vi "VI Server_Set Signaling Control Value from String Format_ArrayInput.vi"(6 "Options":T1, 8 "error in (no error)":errorcluster, 9 "Values":string[](array[string]), 10 "Labels":string[](array[string]), 11 "VI Server Cluster":T2={"Labels"=["Label", "Size", "Font", "Heght", "Width", "Ledding Denominator", "Ledding Nominator", "Label Number", "Microstep Resolution", "X", "Y", "Z", "Italic?", "Underlined?"], "Refs"=[], "VI Ref"=refnum}) -> (0 "error out":errorcluster, 3 "VI Server Cluster.DUP":T2={"Labels"=["Label", "Size", "Font", "Heght", "Width", "Ledding Denominator", "Ledding Nominator", "Label Number", "Microstep Resolution", "X", "Y", "Z", "Italic?", "Underlined?"], "Refs"=[], "VI Ref"=refnum}, 5 "FailedLabel":string)   [LabVIEW 2020]
doc: "<B>Set Control Values From String Formats.vi</B> and converts string values of the selected GUI objects onto original data type."
uses:
  VI Server_TypeDefs/VI Server_RefsCluster.ctl
  VI Server Libraries/VI Server Controls.llb/VI Server_GetSet Controls From String Format_Options.ctl
  <vilib>/userDefined/High Color/IMAQdx.ctl
  VI Server Toolkit LV2013.lvlib
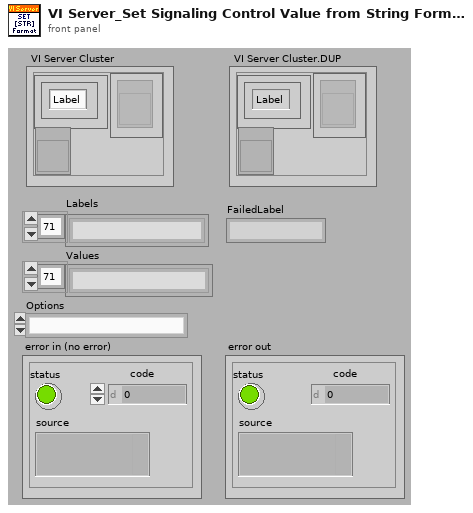
[diagram p1: front panel]
types:
  T1 = typedef "VI Server Toolkit LV2013.lvlib/VI Server_GetSet Controls From String Format_Options.ctl" = enum16{"", "If Ring Get Selection", "If Ring Set by Selection"}
  T2 = typedef "VI Server_RefsCluster.ctl" = cluster{"Labels":string[], "Refs":refnum<vi>[], "VI Ref":refnum<vi>}
  T3 = typedef "IMAQdx.ctl" = refnum<k21>
  T4 = typedef "LVStringsAndValuesArrayTypeDef_U32.ctl" = cluster{"String":string, "Value":u32}[]
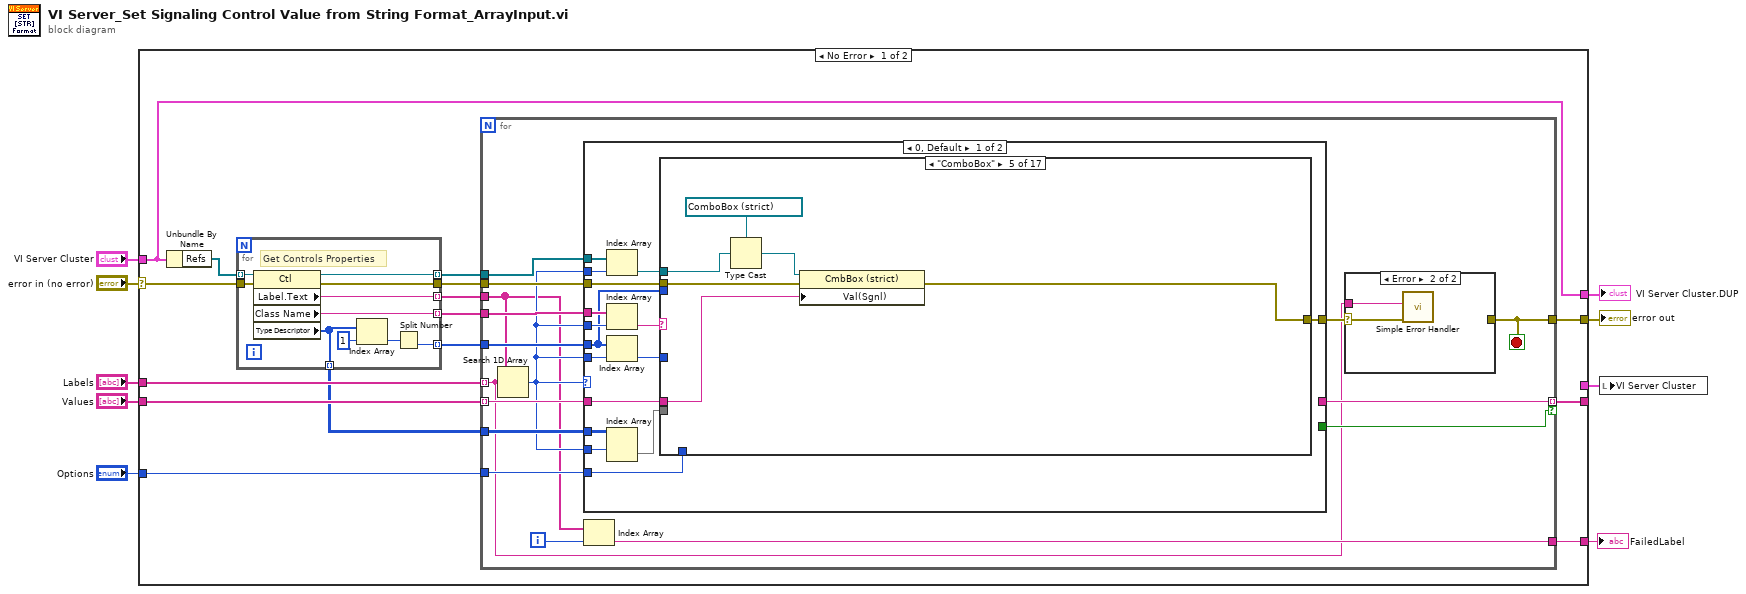
[diagram p0: block diagram]
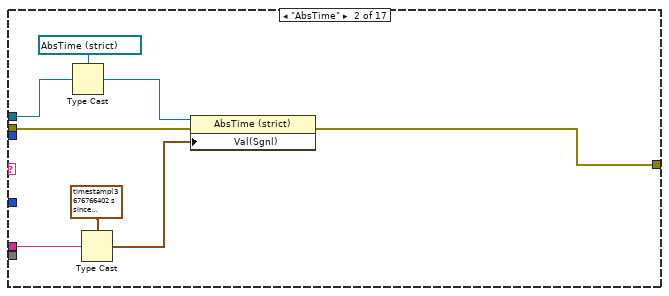
[diagram p4: hidden frame]
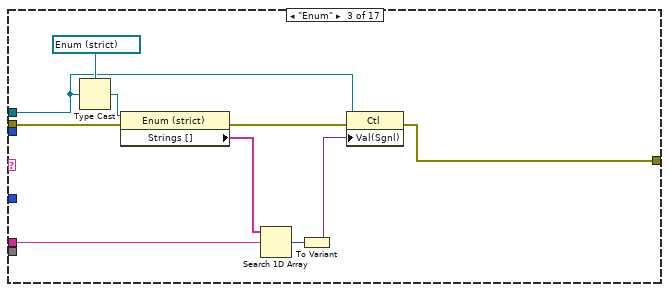
[diagram p5: hidden frame]
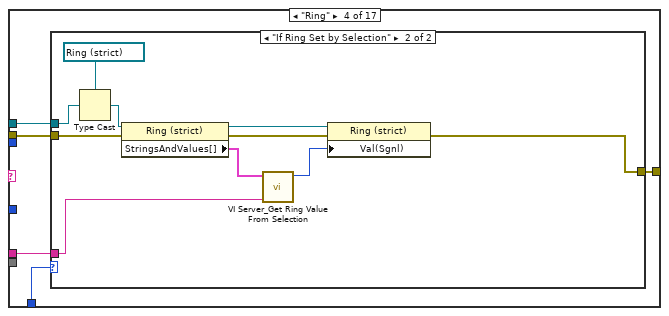
[diagram p6: hidden frame]
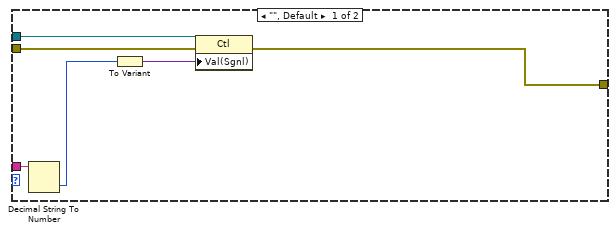
[diagram p7: hidden frame]
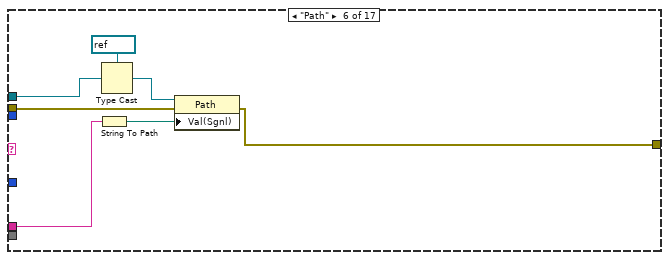
[diagram p8: hidden frame]
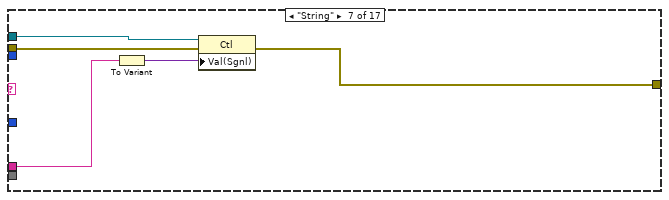
[diagram p9: hidden frame]
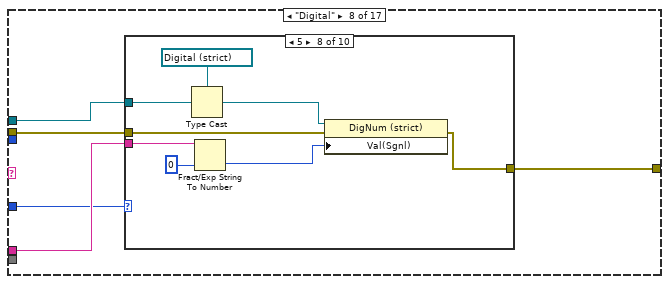
[diagram p10: hidden frame]
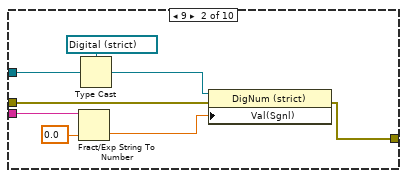
[diagram p12: hidden frame]
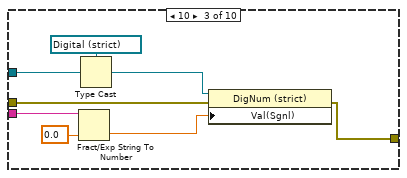
[diagram p13: hidden frame]
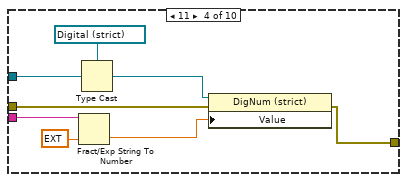
[diagram p14: hidden frame]
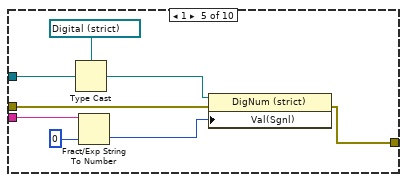
[diagram p15: hidden frame]
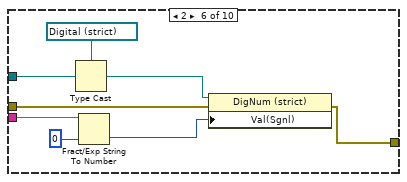
[diagram p16: hidden frame]
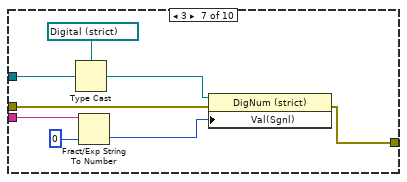
[diagram p17: hidden frame]
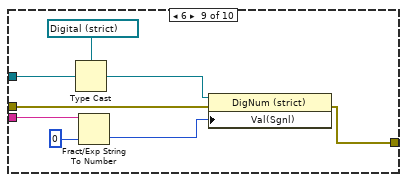
[diagram p18: hidden frame]
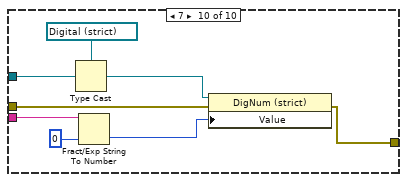
[diagram p19: hidden frame]
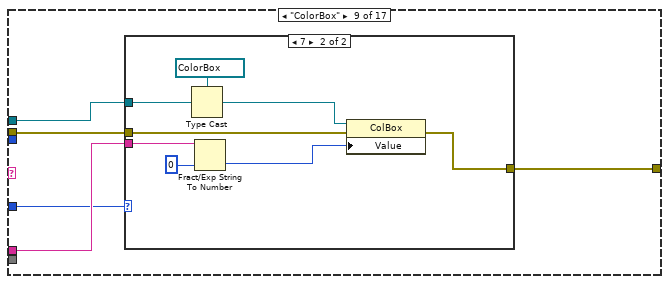
[diagram p20: hidden frame]
diagram:
  n1 = case shown="No Error" "error in (no error)" {
    selector: "error in (no error)" -> [w14 w631]
    tunnel: "Labels" -> [w19 _]
    tunnel: "Values" -> [w20 _]
    tunnel: [w13 w631] -> w7
    tunnel: [w12 _] -> w5
    tunnel: "VI Server Cluster" -> [w12 _]
    tunnel: "Options" -> [w15 _]
    tunnel: [_ w630] -> w2
    tunnel: [w11 _] -> _
    tunnel: [w10 _] -> w1
    frame No Error {
      n2 = Unbundle By Name(w12) -> ("Refs"=w18:refnum<vi>[])
      n3 = for {
        tunnel: w18 -> [w629] mode=indexing
        tunnel: w14 -> [w628]
        tunnel: [w627] -> w24 mode=indexing
        tunnel: [w626] -> w22 mode=indexing
        tunnel: [w625] -> w23 mode=indexing
        tunnel: [w624] -> w21
        tunnel: [w621] -> w17 mode=indexing
        tunnel: [w620] -> w16 mode=indexing
        # "Get Controls Properties"
        n4 = property class="Ctl"(reference=w629, error in=w628) -> (reference out=w625:refnum<vi>, error out=w624:errorcluster, "Label.Text"=w627:string, "Class Name"=w626:string, "Type Descriptor"=w620:i16[])
        n5 = Index Array(array=w620, index=1) -> (element=w622:i16)
        n6 = Split Number(x=w622) -> (lo(x)=w621:u8)  [unwired: 1 out]
      }
      n7 = for {
        tunnel: w19 -> [w25] mode=indexing
        tunnel: w24 -> [w30]
        tunnel: w23 -> [w38]
        tunnel: w22 -> [w40]
        tunnel: w20 -> [w39] mode=indexing
        tunnel: w21 -> [w37]
        tunnel: [w26] -> w13
        tunnel: w17 -> [w36]
        tunnel: w16 -> [w35]
        tunnel: w15 -> [w33]
        tunnel: [w32] -> w11 mode=indexing if=w31
        tunnel: [w28] -> w10
        i -> [w29]
        stop <- w26 stop-if-true
        n8 = Search 1D Array(1D array=w30, element=w25) -> (index of element=w34:i32)  [unwired: 1 out]
        n9 = case shown="0, Default" w34 {
          tunnel: w38 -> [w59 _]
          tunnel: w34 -> [w58 _]
          tunnel: w40 -> [w57 _]
          tunnel: w34 -> [w56 _]
          tunnel: w39 -> [w53 w618]
          tunnel: w37 -> [w52 w619]
          tunnel: [w51 w619] -> w27
          tunnel: w36 -> [w48 _]
          tunnel: w34 -> [w50 _]
          tunnel: w35 -> [w46 _]
          tunnel: w34 -> [w47 _]
          tunnel: w33 -> [w44 _]
          tunnel: [_ w618] -> w32
          tunnel: [_ TRUE] -> w31
          frame 0, Default {
            n10 = Index Array(array=w59, index=w58) -> (element=w54:refnum<vi>)
            n11 = Index Array(array=w57, index=w56) -> (element=w55:string)
            n12 = Index Array(array=w48, index=w50) -> (element=w49:u8)
            n13 = Index Array(array=w46, index (row)=w47) -> (element=w45:i16[])  [unwired: 1 in]
            n14 = case shown="\"ComboBox\"" w55 {
              tunnel: w54 -> [_ w68 w71 w80 w103 w108 w117 w120 w198 w212 w302 w309 w316 w488 w510 w531 w537]
              tunnel: w53 -> [_ w66 w76 w83 w100 w111 w115 w119 w197 w211 w295 w307 w315 w486 w511 w532 w538]
              tunnel: w52 -> [w60 w64 w74 w82 w105 w109 w114 w122 w200 w214 w304 w310 w320 w490 w512 w526 w539]
              tunnel: [w60 w63 w72 w81 w104 w110 w113 w121 w199 w213 w303 w305 w319 w489 w509 w529 w536] -> w51
              tunnel: w49 -> [_ _ _ _ _ _ _ w118 w196 w210 _ _ _ w487 _ _ _]
              tunnel: w48 -> [_ _ _ _ _ _ _ _ _ _ _ _ _ _ _ _ _]
              tunnel: w45 -> [_ _ _ _ _ _ _ _ _ _ _ _ w318 _ _ _ w535]
              tunnel: w44 -> [_ _ _ w79 _ _ _ _ _ _ _ _ _ _ _ _ _]
              frame "", Default {
              }
              frame "AbsTime" {
                n15 = Type Cast(type=refnum<vi> refnum ("UtilizationData.From"), x=w68) -> (*(type *) &x=w62:refnum<vi>)
                n16 = Type Cast(type=timestamp(3676766402.6552744 s since 1904-01-01) ("UtilizationData.From"), x=w66) -> (*(type *) &x=w61:timestamp)
                n17 = property class="AbsTime (strict)"(reference=w62, error in=w64, "Val(Sgnl)"=w61) -> (error out=w63:errorcluster)  [unwired: 1 out]
              }
              frame "Enum" {
                n18 = Type Cast(type=refnum<vi> refnum ("Enum"), x=w71) -> (*(type *) &x=w77:refnum<vi>)
                n19 = property class="Enum (strict)"(reference=w77, error in=w74) -> (error out=w73:errorcluster, "Strings []"=w75:string[])  [unwired: 1 out]
                n20 = Search 1D Array(1D array=w75, element=w76) -> (index of element=w70:i32)  [unwired: 1 out]
                n21 = To Variant(anything=w70) -> (Variant=w69:variant)
                n22 = property class="Ctl"(reference=w71, error in=w73, "Val(Sgnl)"=w69) -> (error out=w72:errorcluster)  [unwired: 1 out]
              }
              frame "Ring" {
                n23 = case shown="\"If Ring Set by Selection\"" w79 {
                  tunnel: w83 -> [w87 w93]
                  tunnel: w82 -> [w89 w98]
                  tunnel: [w88 w96] -> w81
                  tunnel: w80 -> [w85 w95]
                  frame "", Default {
                    n24 = Decimal String To Number(string=w87) -> (number=w86:i32)  [unwired: 2 in, 1 out]
                    n25 = To Variant(anything=w86) -> (Variant=w84:variant)
                    n26 = property class="Ctl"(reference=w85, error in=w89, "Val(Sgnl)"=w84) -> (error out=w88:errorcluster)  [unwired: 1 out]
                  }
                  frame "If Ring Set by Selection" {
                    n27 = Type Cast(type=refnum<vi> refnum ("C-867.SerialPort.Baud Rate"), x=w95) -> (*(type *) &x=w99:refnum<vi>)
                    n28 = property class="Ring (strict)"(reference=w99, error in=w98) -> (reference out=w92:refnum<vi>, error out=w97:errorcluster, "StringsAndValues[]"=w94:T4)
                    n29 = call "VI Server_Get Ring Value From Selection.vi"("Item.Selected"=w93, "StringsAndValues[]"=w94) -> ("Value"=w91:u32)  [unwired: 9 in]
                    n30 = property class="Ring (strict)"(reference=w92, error in=w97, "Val(Sgnl)"=w91) -> (error out=w96:errorcluster)  [unwired: 1 out]
                  }
                }
              }
              frame "ComboBox" {
                n31 = Type Cast(type=refnum<vi> refnum ("OS.SelectChannel"), x=w103) -> (*(type *) &x=w102:refnum<vi>)
                n32 = property class="CmbBox (strict)"(reference=w102, error in=w105, "Val(Sgnl)"=w100) -> (error out=w104:errorcluster)  [unwired: 1 out]
              }
              frame "Path" {
                n33 = String To Path(string=w111) -> (path=w112:path)
                n34 = Type Cast(type=refnum<vi> refnum ("Path"), x=w108) -> (*(type *) &x=w107:refnum<vi>)
                n35 = property class="Path"(reference=w107, error in=w109, "Val(Sgnl)"=w112) -> (error out=w110:errorcluster)  [unwired: 1 out]
              }
              frame "String" {
                n36 = To Variant(anything=w115) -> (Variant=w116:variant)
                n37 = property class="Ctl"(reference=w117, error in=w114, "Val(Sgnl)"=w116) -> (error out=w113:errorcluster)  [unwired: 1 out]
              }
              frame "Digital" {
                n38 = case shown="5" w118 {
                  tunnel: w122 -> [w123 w131 w139 w147 w155 w163 w171 w179 w187 w195]
                  tunnel: [w123 w130 w138 w146 w154 w162 w170 w178 w186 w194] -> w121
                  tunnel: w120 -> [_ w129 w137 w145 w153 w161 w169 w177 w185 w193]
                  tunnel: w119 -> [_ w127 w134 w143 w151 w159 w167 w175 w183 w191]
                  frame 0, Default {
                  }
                  frame 9 {
                    n39 = Fract/Exp String To Number(string=w127, default (0 dbl)=sgl 0.0) -> (number=w126:sgl)  [unwired: 3 out]
                    n40 = Type Cast(type=refnum<vi> refnum ("SGL"), x=w129) -> (*(type *) &x=w128:refnum<vi>)
                    n41 = property class="DigNum (strict)"(reference=w128, error in=w131, "Val(Sgnl)"=w126) -> (error out=w130:errorcluster)  [unwired: 1 out]
                  }
                  frame 10 {
                    n42 = Fract/Exp String To Number(string=w134, default (0 dbl)=0.0) -> (number=w133:dbl)  [unwired: 3 out]
                    n43 = Type Cast(type=refnum<vi> refnum ("DBL"), x=w137) -> (*(type *) &x=w135:refnum<vi>)
                    n44 = property class="DigNum (strict)"(reference=w135, error in=w139, "Val(Sgnl)"=w133) -> (error out=w138:errorcluster)  [unwired: 1 out]
                  }
                  frame 11 {
                    n45 = Fract/Exp String To Number(string=w143, default (0 dbl)=ext 0.0) -> (number=w142:ext)  [unwired: 3 out]
                    n46 = Type Cast(type=refnum<vi> refnum ("EXT"), x=w145) -> (*(type *) &x=w144:refnum<vi>)
                    n47 = property class="DigNum (strict)"(reference=w144, error in=w147, "Value"=w142) -> (error out=w146:errorcluster)  [unwired: 1 out]
                  }
                  frame 1 {
                    n48 = Type Cast(type=refnum<vi> refnum ("I8"), x=w153) -> (*(type *) &x=w152:refnum<vi>)
                    n49 = Fract/Exp String To Number(string=w151, default (0 dbl)=i8 0) -> (number=w150:i8)  [unwired: 3 out]
                    n50 = property class="DigNum (strict)"(reference=w152, error in=w155, "Val(Sgnl)"=w150) -> (error out=w154:errorcluster)  [unwired: 1 out]
                  }
                  frame 2 {
                    n51 = Type Cast(type=refnum<vi> refnum ("I16"), x=w161) -> (*(type *) &x=w160:refnum<vi>)
                    n52 = Fract/Exp String To Number(string=w159, default (0 dbl)=i16 0) -> (number=w158:i16)  [unwired: 3 out]
                    n53 = property class="DigNum (strict)"(reference=w160, error in=w163, "Val(Sgnl)"=w158) -> (error out=w162:errorcluster)  [unwired: 1 out]
                  }
                  frame 3 {
                    n54 = Type Cast(type=refnum<vi> refnum ("I32"), x=w169) -> (*(type *) &x=w168:refnum<vi>)
                    n55 = Fract/Exp String To Number(string=w167, default (0 dbl)=0) -> (number=w166:i32)  [unwired: 3 out]
                    n56 = property class="DigNum (strict)"(reference=w168, error in=w171, "Val(Sgnl)"=w166) -> (error out=w170:errorcluster)  [unwired: 1 out]
                  }
                  frame 5 {
                    n57 = Type Cast(type=refnum<vi> refnum ("U8"), x=w177) -> (*(type *) &x=w176:refnum<vi>)
                    n58 = Fract/Exp String To Number(string=w175, default (0 dbl)=u8 0) -> (number=w174:u8)  [unwired: 3 out]
                    n59 = property class="DigNum (strict)"(reference=w176, error in=w179, "Val(Sgnl)"=w174) -> (error out=w178:errorcluster)  [unwired: 1 out]
                  }
                  frame 6 {
                    n60 = Type Cast(type=refnum<vi> refnum ("U16"), x=w185) -> (*(type *) &x=w184:refnum<vi>)
                    n61 = Fract/Exp String To Number(string=w183, default (0 dbl)=u16 0) -> (number=w182:u16)  [unwired: 3 out]
                    n62 = property class="DigNum (strict)"(reference=w184, error in=w187, "Val(Sgnl)"=w182) -> (error out=w186:errorcluster)  [unwired: 1 out]
                  }
                  frame 7 {
                    n63 = Type Cast(type=refnum<vi> refnum ("U32"), x=w193) -> (*(type *) &x=w192:refnum<vi>)
                    n64 = Fract/Exp String To Number(string=w191, default (0 dbl)=u32 0) -> (number=w190:u32)  [unwired: 3 out]
                    n65 = property class="DigNum (strict)"(reference=w192, error in=w195, "Value"=w190) -> (error out=w194:errorcluster)  [unwired: 1 out]
                  }
                }
              }
              frame "ColorBox" {
                n66 = case shown="7" w196 {
                  tunnel: w200 -> [w201 w209]
                  tunnel: [w201 w208] -> w199
                  tunnel: w198 -> [_ w207]
                  tunnel: w197 -> [_ w205]
                  frame 0, Default {
                  }
                  frame 7 {
                    n67 = Type Cast(type=refnum<vi> refnum ("Limits.RPM.Scale.Color<=1000"), x=w207) -> (*(type *) &x=w206:refnum<vi>)
                    n68 = Fract/Exp String To Number(string=w205, default (0 dbl)=u32 0) -> (number=w204:u32)  [unwired: 3 out]
                    n69 = property class="ColBox"(reference=w206, error in=w209, "Value"=w204) -> (error out=w208:errorcluster)  [unwired: 1 out]
                  }
                }
              }
              frame "Slide" {
                n70 = case shown="7" w210 {
                  tunnel: w214 -> [w215 w223 w232 w241 w249 w257 w265 w273 w281 w289]
                  tunnel: [w215 w222 w231 w240 w248 w256 w264 w272 w280 w288] -> w213
                  tunnel: w212 -> [_ w221 w230 w239 w247 w255 w263 w271 w279 w287]
                  tunnel: w211 -> [_ w219 w227 w237 w245 w253 w261 w269 w277 w285]
                  frame 0, Default {
                  }
                  frame 9 {
                    n71 = Fract/Exp String To Number(string=w219, default (0 dbl)=sgl 0.0) -> (number=w218:sgl)  [unwired: 3 out]
                    n72 = Type Cast(type=refnum<vi> refnum ("SGL 2"), x=w221) -> (*(type *) &x=w220:refnum<vi>)
                    n73 = property class="DigNum (strict)"(reference=w220, error in=w223, "Value"=w218) -> (reference out=w224:refnum<vi>, error out=w222:errorcluster)
                    n74 = Close Reference(reference=w224) -> ()  [unwired: 1 in, 1 out]
                  }
                  frame 10 {
                    n75 = Fract/Exp String To Number(string=w227, default (0 dbl)=0.0) -> (number=w226:dbl)  [unwired: 3 out]
                    n76 = Type Cast(type=refnum<vi> refnum ("DBL 2"), x=w230) -> (*(type *) &x=w228:refnum<vi>)
                    n77 = property class="DigNum (strict)"(reference=w228, error in=w232, "Val(Sgnl)"=w226) -> (reference out=w233:refnum<vi>, error out=w231:errorcluster)
                    n78 = Close Reference(reference=w233) -> ()  [unwired: 1 in, 1 out]
                  }
                  frame 11 {
                    n79 = Fract/Exp String To Number(string=w237, default (0 dbl)=ext 0.0) -> (number=w236:ext)  [unwired: 3 out]
                    n80 = Type Cast(type=refnum<vi> refnum ("EXT 2"), x=w239) -> (*(type *) &x=w238:refnum<vi>)
                    n81 = property class="DigNum (strict)"(reference=w238, error in=w241, "Val(Sgnl)"=w236) -> (error out=w240:errorcluster)  [unwired: 1 out]
                  }
                  frame 1 {
                    n82 = Type Cast(type=refnum<vi> refnum ("I8 2"), x=w247) -> (*(type *) &x=w246:refnum<vi>)
                    n83 = Fract/Exp String To Number(string=w245, default (0 dbl)=i8 0) -> (number=w244:i8)  [unwired: 3 out]
                    n84 = property class="DigNum (strict)"(reference=w246, error in=w249, "Val(Sgnl)"=w244) -> (error out=w248:errorcluster)  [unwired: 1 out]
                  }
                  frame 2 {
                    n85 = Type Cast(type=refnum<vi> refnum ("I16 2"), x=w255) -> (*(type *) &x=w254:refnum<vi>)
                    n86 = Fract/Exp String To Number(string=w253, default (0 dbl)=i16 0) -> (number=w252:i16)  [unwired: 3 out]
                    n87 = property class="DigNum (strict)"(reference=w254, error in=w257, "Value"=w252) -> (error out=w256:errorcluster)  [unwired: 1 out]
                  }
                  frame 3 {
                    n88 = Type Cast(type=refnum<vi> refnum ("I32 2"), x=w263) -> (*(type *) &x=w262:refnum<vi>)
                    n89 = Fract/Exp String To Number(string=w261, default (0 dbl)=0) -> (number=w260:i32)  [unwired: 3 out]
                    n90 = property class="DigNum (strict)"(reference=w262, error in=w265, "Val(Sgnl)"=w260) -> (error out=w264:errorcluster)  [unwired: 1 out]
                  }
                  frame 5 {
                    n91 = Type Cast(type=refnum<vi> refnum ("U8 2"), x=w271) -> (*(type *) &x=w270:refnum<vi>)
                    n92 = Fract/Exp String To Number(string=w269, default (0 dbl)=u8 0) -> (number=w268:u8)  [unwired: 3 out]
                    n93 = property class="DigNum (strict)"(reference=w270, error in=w273, "Value"=w268) -> (error out=w272:errorcluster)  [unwired: 1 out]
                  }
                  frame 6 {
                    n94 = Type Cast(type=refnum<vi> refnum ("U16 2"), x=w279) -> (*(type *) &x=w278:refnum<vi>)
                    n95 = Fract/Exp String To Number(string=w277, default (0 dbl)=u16 0) -> (number=w276:u16)  [unwired: 3 out]
                    n96 = property class="DigNum (strict)"(reference=w278, error in=w281, "Val(Sgnl)"=w276) -> (error out=w280:errorcluster)  [unwired: 1 out]
                  }
                  frame 7 {
                    n97 = Type Cast(type=refnum<vi> refnum ("U32 2"), x=w287) -> (*(type *) &x=w286:refnum<vi>)
                    n98 = Fract/Exp String To Number(string=w285, default (0 dbl)=u32 0) -> (number=w284:u32)  [unwired: 3 out]
                    n99 = property class="DigNum (strict)"(reference=w286, error in=w289, "Val(Sgnl)"=w284) -> (error out=w288:errorcluster)  [unwired: 1 out]
                  }
                }
              }
              frame "Boolean" {
                n100 = Type Cast(type=refnum<vi> refnum ("Boolean"), x=w302) -> (*(type *) &x=w300:refnum<vi>)
                n101 = Equal?(x=w295, y="TRUE" ("x")) -> (x = y?=w298:bool)
                n102 = Equal?(x=w295, y="ON" ("x")) -> (x = y?=w294:bool)
                n103 = Equal?(x=w295, y="1" ("x")) -> (x = y?=w293:bool)
                n104 = Compound Arithmetic op=OR(w298, w294, w293) -> (w292:bool)
                n105 = Type Cast(type=FALSE ("Value"), x=w292) -> (*(type *) &x=w290:bool)
                n106 = property class="Bool (strict)"(reference=w300, error in=w304, "Val(Sgnl)"=w290) -> (error out=w303:errorcluster)  [unwired: 1 out]
              }
              frame "Table" {
                n107 = Type Cast(type=refnum<vi> refnum ("Image Statistics Table"), x=w309) -> (*(type *) &x=w312:refnum<vi>)
                n108 = Spreadsheet String To Array(delimiter (Tab)=",", format string="%s", spreadsheet string=w307, array type (2D Dbl)=string[][] []) -> (array=w306:string[][])
                n109 = property class="Tbl (strict)"(reference=w312, error in=w310, "Val(Sgnl)"=w306) -> (error out=w305:errorcluster)  [unwired: 1 out]
              }
              frame "Array" {
                n110 = Index Array(array=w318, index=2) -> (element=w317:i16)
                n111 = case shown="1" w317 {
                  tunnel: w318 -> [_ w328 w370]
                  tunnel: w320 -> [w322 w327 w369]
                  tunnel: [w322 w325 w368] -> w319
                  tunnel: w316 -> [_ w324 w367]
                  tunnel: w315 -> [_ w323 w366]
                  frame 0, Default {
                  }
                  frame 1 {
                    # "1D Array\ndata Type"
                    n112 = Index Array(array=w328, index=6) -> (element=w326:i16)
                    n113 = case shown="4032" w326 {
                      tunnel: w324 -> [_ w340 w350 w361]
                      tunnel: [w330 w338 w348 w359] -> w325
                      tunnel: w327 -> [w330 w337 w347 w358]
                      tunnel: w323 -> [_ w333 w343 w356]
                      frame 0, Default {
                      }
                      frame 16394 {
                        n114 = Spreadsheet String To Array(delimiter (Tab)=",", format string="%0.6f", spreadsheet string=w333, array type (2D Dbl)=dbl[] []) -> (array=w331:dbl[])
                        n115 = Type Cast(type=refnum<vi> refnum ("Array"), x=w340) -> (*(type *) &x=w339:refnum<vi>)
                        n116 = property class="Arr (strict)"(reference=w339, error in=w337, "Val(Sgnl)"=w331) -> (error out=w338:errorcluster)  [unwired: 1 out]
                      }
                      frame 16432 {
                        n117 = Spreadsheet String To Array(delimiter (Tab)=",", format string="%s", spreadsheet string=w343, array type (2D Dbl)=string[] []) -> (array=w341:string[])
                        n118 = Type Cast(type=refnum<vi> refnum ("1D String"), x=w350) -> (*(type *) &x=w349:refnum<vi>)
                        n119 = property class="Arr (strict)"(reference=w349, error in=w347, "Val(Sgnl)"=w341) -> (error out=w348:errorcluster)  [unwired: 1 out]
                      }
                      frame 16434 {
                        n120 = Spreadsheet String To Array(delimiter (Tab)=",", format string="%s", spreadsheet string=w356, array type (2D Dbl)=string[] []) -> (array=w352:string[])
                        n121 = for {
                          tunnel: w352 -> [w363] mode=indexing
                          tunnel: [w362] -> w351 mode=indexing
                          n122 = String To Path(string=w363) -> (path=w362:path)
                        }
                        n123 = Type Cast(type=refnum<vi> refnum ("Array"), x=w361) -> (*(type *) &x=w360:refnum<vi>)
                        n124 = property class="Arr (strict)"(reference=w360, error in=w358, "Val(Sgnl)"=w351) -> (error out=w359:errorcluster)  [unwired: 1 out]
                      }
                    }
                  }
                  frame 2 {
                    n125 = Index Array(array=w370, index=8) -> (element=w365:i16)
                    n126 = Split Number(x=w365) -> (lo(x)=w364:u8)  [unwired: 1 out]
                    n127 = case shown="32" w364 {
                      tunnel: w367 -> [_ w382 w392 w402 w412 w422 w432 w442 w452 w462 w472 w483]
                      tunnel: [w372 w380 w390 w400 w410 w420 w430 w440 w450 w460 w470 w481] -> w368
                      tunnel: w369 -> [w372 w379 w389 w399 w409 w419 w429 w439 w449 w459 w469 w480]
                      tunnel: w366 -> [_ w376 w386 w396 w406 w416 w426 w436 w446 w456 w466 w479]
                      frame 0, Default {
                      }
                      frame 1 {
                        n128 = Spreadsheet String To Array(delimiter (Tab)=",", format string="%d", spreadsheet string=w376, array type (2D Dbl)=i8[][] []) -> (array=w374:i8[][])
                        n129 = Type Cast(type=refnum<vi> refnum ("Array"), x=w382) -> (*(type *) &x=w381:refnum<vi>)
                        n130 = property class="Arr (strict)"(reference=w381, error in=w379, "Val(Sgnl)"=w374) -> (error out=w380:errorcluster)  [unwired: 1 out]
                      }
                      frame 2 {
                        n131 = Spreadsheet String To Array(delimiter (Tab)=",", format string="%d", spreadsheet string=w386, array type (2D Dbl)=i16[][] []) -> (array=w384:i16[][])
                        n132 = Type Cast(type=refnum<vi> refnum ("Array"), x=w392) -> (*(type *) &x=w391:refnum<vi>)
                        n133 = property class="Arr (strict)"(reference=w391, error in=w389, "Val(Sgnl)"=w384) -> (error out=w390:errorcluster)  [unwired: 1 out]
                      }
                      frame 3 {
                        n134 = Spreadsheet String To Array(delimiter (Tab)=",", format string="%d", spreadsheet string=w396, array type (2D Dbl)=i32[][] []) -> (array=w394:i32[][])
                        n135 = Type Cast(type=refnum<vi> refnum ("Array"), x=w402) -> (*(type *) &x=w401:refnum<vi>)
                        n136 = property class="Arr (strict)"(reference=w401, error in=w399, "Val(Sgnl)"=w394) -> (error out=w400:errorcluster)  [unwired: 1 out]
                      }
                      frame 5 {
                        n137 = Spreadsheet String To Array(delimiter (Tab)=",", format string="%d", spreadsheet string=w406, array type (2D Dbl)=u8[][] []) -> (array=w404:u8[][])
                        n138 = Type Cast(type=refnum<vi> refnum ("Array"), x=w412) -> (*(type *) &x=w411:refnum<vi>)
                        n139 = property class="Arr (strict)"(reference=w411, error in=w409, "Val(Sgnl)"=w404) -> (error out=w410:errorcluster)  [unwired: 1 out]
                      }
                      frame 6 {
                        n140 = Spreadsheet String To Array(delimiter (Tab)=",", format string="%d", spreadsheet string=w416, array type (2D Dbl)=u16[][] []) -> (array=w414:u16[][])
                        n141 = Type Cast(type=refnum<vi> refnum ("Array"), x=w422) -> (*(type *) &x=w421:refnum<vi>)
                        n142 = property class="Arr (strict)"(reference=w421, error in=w419, "Val(Sgnl)"=w414) -> (error out=w420:errorcluster)  [unwired: 1 out]
                      }
                      frame 7 {
                        n143 = Spreadsheet String To Array(delimiter (Tab)=",", format string="%d", spreadsheet string=w426, array type (2D Dbl)=u32[][] []) -> (array=w424:u32[][])
                        n144 = Type Cast(type=refnum<vi> refnum ("Array"), x=w432) -> (*(type *) &x=w431:refnum<vi>)
                        n145 = property class="Arr (strict)"(reference=w431, error in=w429, "Val(Sgnl)"=w424) -> (error out=w430:errorcluster)  [unwired: 1 out]
                      }
                      frame 9 {
                        n146 = Spreadsheet String To Array(delimiter (Tab)=",", format string="%f", spreadsheet string=w436, array type (2D Dbl)=sgl[][] []) -> (array=w434:sgl[][])
                        n147 = Type Cast(type=refnum<vi> refnum ("Array"), x=w442) -> (*(type *) &x=w441:refnum<vi>)
                        n148 = property class="Arr (strict)"(reference=w441, error in=w439, "Val(Sgnl)"=w434) -> (error out=w440:errorcluster)  [unwired: 1 out]
                      }
                      frame 10 {
                        n149 = Spreadsheet String To Array(delimiter (Tab)=",", format string="%f", spreadsheet string=w446, array type (2D Dbl)=dbl[][] []) -> (array=w444:dbl[][])
                        n150 = Type Cast(type=refnum<vi> refnum ("Array"), x=w452) -> (*(type *) &x=w451:refnum<vi>)
                        n151 = property class="Arr (strict)"(reference=w451, error in=w449, "Val(Sgnl)"=w444) -> (error out=w450:errorcluster)  [unwired: 1 out]
                      }
                      frame 11 {
                        n152 = Spreadsheet String To Array(delimiter (Tab)=",", format string="%f", spreadsheet string=w456, array type (2D Dbl)=ext[][] []) -> (array=w454:ext[][])
                        n153 = Type Cast(type=refnum<vi> refnum ("Array"), x=w462) -> (*(type *) &x=w461:refnum<vi>)
                        n154 = property class="Arr (strict)"(reference=w461, error in=w459, "Val(Sgnl)"=w454) -> (error out=w460:errorcluster)  [unwired: 1 out]
                      }
                      frame 48 {
                        n155 = Spreadsheet String To Array(delimiter (Tab)=",", format string="%s", spreadsheet string=w466, array type (2D Dbl)=string[][] []) -> (array=w464:string[][])
                        n156 = Type Cast(type=refnum<vi> refnum ("Array"), x=w472) -> (*(type *) &x=w471:refnum<vi>)
                        n157 = property class="Arr (strict)"(reference=w471, error in=w469, "Val(Sgnl)"=w464) -> (error out=w470:errorcluster)  [unwired: 1 out]
                      }
                      frame 50 {
                        n158 = Spreadsheet String To Array(delimiter (Tab)=",", format string="%s", spreadsheet string=w479, array type (2D Dbl)=string[][] []) -> (array=w475:string[][])
                        n159 = for {
                          tunnel: w475 -> [w485] mode=indexing
                          tunnel: [w484] -> w474 mode=indexing
                          n160 = String To Path(string=w485) -> (path=w484:path[])
                        }
                        n161 = Type Cast(type=refnum<vi> refnum ("Array"), x=w483) -> (*(type *) &x=w482:refnum<vi>)
                        n162 = property class="Arr (strict)"(reference=w482, error in=w480, "Val(Sgnl)"=w474) -> (error out=w481:errorcluster)  [unwired: 1 out]
                      }
                    }
                  }
                }
              }
              frame "MulticolumnListbox" {
                n163 = case shown="3" w487 {
                  tunnel: w490 -> [w491 w496 w507]
                  tunnel: [w491 w495 w506] -> w489
                  tunnel: w488 -> [_ w498 w508]
                  tunnel: w486 -> [_ w493 w503]
                  frame 0, Default {
                  }
                  frame 3 {
                    n164 = Decimal String To Number(string=w493) -> (number=w492:i32)  [unwired: 2 in, 1 out]
                    n165 = Type Cast(type=refnum<vi> refnum ("Controls Description"), x=w498) -> (*(type *) &x=w494:refnum<vi>)
                    n166 = property class="MCListbox (strict)"(reference=w494, error in=w496, "Val(Sgnl)"=w492) -> (error out=w495:errorcluster)  [unwired: 1 out]
                  }
                  frame 64 {
                    n167 = Spreadsheet String To Array(delimiter (Tab)=",", format string="%s", spreadsheet string=w503, array type (2D Dbl)=i32[] [] ("Value")) -> (array=w499:i32[])
                    n168 = Type Cast(type=refnum<vi> refnum ("Controls Description"), x=w508) -> (*(type *) &x=w505:refnum<vi>)
                    n169 = property class="MCListbox (strict)"(reference=w505, error in=w507, "Val(Sgnl)"=w499) -> (error out=w506:errorcluster)  [unwired: 1 out]
                  }
                }
              }
              frame "GenClassTagRef" {
                n170 = disable-structure shown="Disabled" {
                  disable-tunnel: w512 -> [w522 w523]
                  disable-tunnel: w511 -> [w521 _]
                  disable-tunnel: w510 -> [w519 _]
                  disable-tunnel: [w514 w523] -> w509
                  frame Disabled {
                    n171 = Type Cast(type=refnum<vi> refnum ("Camera.Left"), x=w519) -> (*(type *) &x=w516:refnum<vi>)
                    n172 = Unflatten From String(type=T3 refnum ("Camera.Left"), binary string=w521, error in (no error)=w522) -> (value=w515:T3, error out=w517:errorcluster)  [unwired: 2 in, 1 out]
                    n173 = property class="IMAQdx (strict)"(reference=w516, error in=w517, "Value"=w515) -> (error out=w513:errorcluster)  [unwired: 1 out]
                    n174 = call <vilib>:"Simple Error Handler.vi"("error in (no error)"=w513) -> ()  [unwired: 4 in, 5 out]
                    n175 = call "Error 74_ClearEmptyFlattenedStringRecovery.vi"("error in"=w513) -> ("error out"=w514:errorcluster)  [unwired: 3 in, 1 out]
                  }
                  frame Enabled {
                  }
                }
              }
              frame "VISAResourceName" {
                n176 = call <vilib>:"Trim Whitespace.vi"("string"=w532) -> ("trimmed string"=w525:string)  [unwired: 1 in]
                n177 = Type Cast(type=refnum<vi> refnum ("VISA resource name"), x=w531) -> (*(type *) &x=w530:refnum<vi>)
                n178 = Type Cast(type=refnum<visa-resource-name> refnum ("GPS.VISA.ResourceName"), x=w525) -> (*(type *) &x=w524:refnum<visa-resource-name>)
                n179 = property class="VISAName"(reference=w530, error in=w526, "Val(Sgnl)"=w524) -> (error out=w529:errorcluster)  [unwired: 1 out]
              }
              frame "DAQmxName" {
                n180 = Index Array(array=w535) -> (element=w534:i16)  [unwired: 1 in]
                n181 = call <vilib>:"Trim Whitespace.vi"("string"=w538) -> ("trimmed string"=w533:string)  [unwired: 1 in]
                n182 = case shown="46" w534 {
                  tunnel: w539 -> [w540 w544 w553 w562 w571 w577 w589 w596 w601 w611]
                  tunnel: w533 -> [_ w542 w552 w560 w569 w579 w588 w595 w604 w613]
                  tunnel: w537 -> [_ w549 w558 w567 w576 w584 w592 w600 w608 w616]
                  tunnel: [w540 w545 w554 w564 w573 w583 w591 w599 w606 w615] -> w536
                  frame 0, Default {
                  }
                  frame 26, 38 {
                    n183 = Type Cast(type=refnum<vi> refnum ("CamTriggerGenerator.Counter"), x=w549) -> (*(type *) &x=w548:refnum<vi>)
                    n184 = Type Cast(type=tag "" ("CamTriggerGenerator.Counter"), x=w542) -> (*(type *) &x=w541:tag)
                    n185 = property class="DAQmxName"(reference=w548, error in=w544, "Value"=w541) -> (error out=w546:errorcluster)  [unwired: 1 out]
                    n186 = call "Error 74_ClearEmptyFlattenedStringRecovery.vi"("error in"=w546) -> ("error out"=w545:errorcluster)  [unwired: 3 in, 1 out]
                  }
                  frame 30 {
                    n187 = Type Cast(type=refnum<vi> refnum ("CamTriggerGenerator.Counter"), x=w558) -> (*(type *) &x=w557:refnum<vi>)
                    n188 = Type Cast(type=tag "Dev2/port1/line3" ("DAQ.GPM.DigitalLine"), x=w552) -> (*(type *) &x=w551:tag)
                    n189 = property class="DAQmxName"(reference=w557, error in=w553, "Value"=w551) -> (error out=w555:errorcluster)  [unwired: 1 out]
                    n190 = call "Error 74_ClearEmptyFlattenedStringRecovery.vi"("error in"=w555) -> ("error out"=w554:errorcluster)  [unwired: 3 in, 1 out]
                  }
                  frame 32 {
                    n191 = Type Cast(type=refnum<vi> refnum ("DAQmx.Digital Output"), x=w567) -> (*(type *) &x=w566:refnum<vi>)
                    n192 = Type Cast(type=tag "" ("DAQmx.Digital Output"), x=w560) -> (*(type *) &x=w561:tag)
                    n193 = property class="DAQmxName"(reference=w566, error in=w562, "Val(Sgnl)"=w561) -> (error out=w565:errorcluster)  [unwired: 1 out]
                    n194 = call "Error 74_ClearEmptyFlattenedStringRecovery.vi"("error in"=w565) -> ("error out"=w564:errorcluster)  [unwired: 3 in, 1 out]
                  }
                  frame 34 {
                    n195 = Type Cast(type=refnum<vi> refnum ("DAQmx.Digital Output"), x=w576) -> (*(type *) &x=w575:refnum<vi>)
                    n196 = Type Cast(type=tag "Dev2/ai1" ("DAQ.EngineTilt.Channel"), x=w569) -> (*(type *) &x=w570:tag)
                    n197 = property class="DAQmxName"(reference=w575, error in=w571, "Val(Sgnl)"=w570) -> (error out=w574:errorcluster)  [unwired: 1 out]
                    n198 = call "Error 74_ClearEmptyFlattenedStringRecovery.vi"("error in"=w574) -> ("error out"=w573:errorcluster)  [unwired: 3 in, 1 out]
                  }
                  frame 40 {
                    n199 = Type Cast(type=refnum<vi> refnum ("IlluminationControl.DigitalLines"), x=w584) -> (*(type *) &x=w582:refnum<vi>)
                    n200 = Type Cast(type=tag "Dev1/ctr0" ("Engine.FuelPump.DAQmx.Counter"), x=w579) -> (*(type *) &x=w578:tag)
                    n201 = property class="DAQmxName"(reference=w582, error in=w577, "Val(Sgnl)"=w578) -> (error out=w583:errorcluster)  [unwired: 1 out]
                  }
                  frame 42, 48 {
                    n202 = Type Cast(type=refnum<vi> refnum ("Engine.FuelPump.PauseTrigger.DO"), x=w592) -> (*(type *) &x=w590:refnum<vi>)
                    n203 = Type Cast(type=tag "Dev1/port0/line7" ("Engine.FuelPump.PauseTrigger.DO"), x=w588) -> (*(type *) &x=w586:tag)
                    n204 = property class="DAQmxName"(reference=w590, error in=w589, "Val(Sgnl)"=w586) -> (error out=w591:errorcluster)  [unwired: 1 out]
                  }
                  frame 44 {
                    n205 = Type Cast(type=refnum<vi> refnum ("IlluminationControl.DigitalLines"), x=w600) -> (*(type *) &x=w598:refnum<vi>)
                    n206 = Type Cast(type=tag "Dev2/port0/line0:1" ("IlluminationControl.DigitalLines"), x=w595) -> (*(type *) &x=w594:tag)
                    n207 = property class="DAQmxName"(reference=w598, error in=w596, "Val(Sgnl)"=w594) -> (error out=w599:errorcluster)  [unwired: 1 out]
                  }
                  frame 46 {
                    n208 = Type Cast(type=refnum<vi> refnum ("Engine.FuelPump.PauseTriggerSource"), x=w608) -> (*(type *) &x=w607:refnum<vi>)
                    n209 = Type Cast(type=tag "Output Terminal" ("CamTriggerGenerator.OutputTerminal"), x=w604) -> (*(type *) &x=w602:tag)
                    n210 = property class="DAQmxName"(reference=w607, error in=w601, "Value"=w602) -> (error out=w606:errorcluster)  [unwired: 1 out]
                  }
                  frame 50 {
                    n211 = Type Cast(type=refnum<vi> refnum ("DAQmx.RPM.FrequencyMonitor.DigitalLine"), x=w616) -> (*(type *) &x=w614:refnum<vi>)
                    n212 = Type Cast(type=tag "" ("DAQmx.RPM.FrequencyMonitor.DigitalLine"), x=w613) -> (*(type *) &x=w612:tag)
                    n213 = property class="DAQmxName"(reference=w614, error in=w611, "Value"=w612) -> (error out=w615:errorcluster)  [unwired: 1 out]
                  }
                }
              }
            }
          }
          frame -1 {
          }
        }
        n214 = Index Array(array=w30, index=w29) -> (element=w28:string)
        n215 = case shown="Error" w27 {
          selector: w27 -> [w41 w43]
          tunnel: [w41 _] -> w26
          tunnel: w25 -> [_ w42]
          frame No Error {
          }
          frame Error {
            n216 = call <vilib>:"Simple Error Handler.vi"("error source (\" \")"=w42, "error in (no error)"=w43) -> ()  [unwired: 3 in, 5 out]
          }
        }
      }
    }
    frame Error {
      n217 = call "VI Server_Empty VI Server Cluster.vi"() -> ("VI Server Cluster"=w630:T2)  [unwired: 7 in]
    }
  }
  "error out" <- w7
  "VI Server Cluster.DUP" <- w5
  "FailedLabel" <- w1
  n218 = local write "VI Server Cluster"(w2) -> ()
